vi "Send SDO.vi"() -> ()   [LabVIEW 2016]
uses:
  <vilib>/CANopenLib/CANOPEN.llb/CANopen SDO Create.vi
  <vilib>/CANopenLib/CANOPEN.llb/CANopen SDO Write [I32].vi
  <vilib>/CANopenLib/CANOPEN.llb/CANopen SDO Read [I32].vi
  <vilib>/CANopenLib/CANOPEN.llb/CANopen SDO Write [I16].vi
  <vilib>/CANopenLib/CANOPEN.llb/CANopen SDO Read [I16].vi
  <vilib>/CANopenLib/CANOPEN.llb/CANopen SDO Write [I8].vi
  <vilib>/CANopenLib/CANOPEN.llb/CANopen SDO Read [I8].vi
  <vilib>/CANopenLib/CANOPEN.llb/CANopen SDO Write [U32].vi
  <vilib>/CANopenLib/CANOPEN.llb/CANopen SDO Read [U32].vi
  <vilib>/CANopenLib/CANOPEN.llb/CANopen SDO Write [U16].vi
  <vilib>/CANopenLib/CANOPEN.llb/CANopen SDO Read [U16].vi
  <vilib>/CANopenLib/CANOPEN.llb/CANopen SDO Write [U8].vi
  <vilib>/CANopenLib/CANOPEN.llb/CANopen SDO Read [U8].vi
  <vilib>/CANopenLib/CANOPEN.llb/CANopen SDO Write [SGL].vi
  <vilib>/CANopenLib/CANOPEN.llb/CANopen SDO Read [SGL].vi
  <vilib>/CANopenLib/CANOPEN.llb/CANopen SDO Write [DBL].vi
  <vilib>/CANopenLib/CANOPEN.llb/CANopen SDO Read [DBL].vi
  <vilib>/CANopenLib/CANOPEN.llb/CANopen SDO Close.vi
  <vilib>/CANopenLib/CANOPEN.llb/CANopen Interface Close.vi
panel:
  out "error online":errorcluster
  in  "client COB-ID (0)":u32
  in  "server COB-ID (0)":u32
  in  "node-ID":u8
  out "error out":errorcluster
  in  "Blank Button 2":bool
  in  "Blank Button":bool
  in  "data":i32
  out "completion code":u32=84148224 format="%.0x"
  out "String":string
  in  "Write?":bool
  in  "object sub-index (0)":u8
  in  "object index":u16 format="%x"
  in  "Menu Ring":u16(ring) items=["u32"=3, "u8"=5]
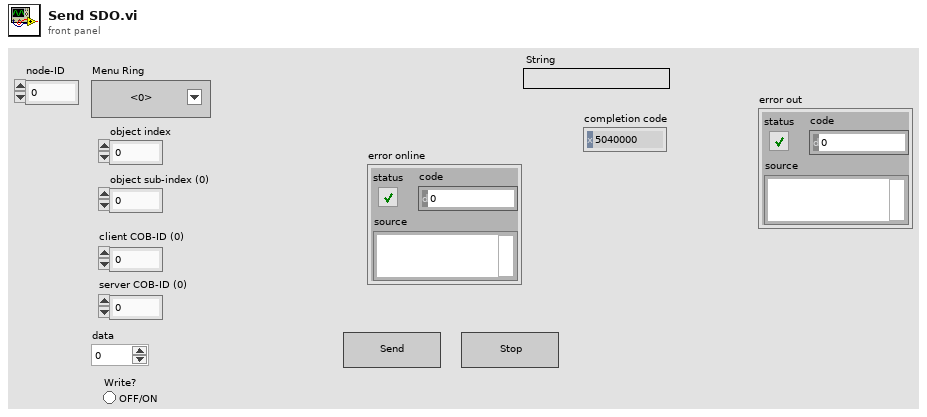
[diagram p1: front panel]
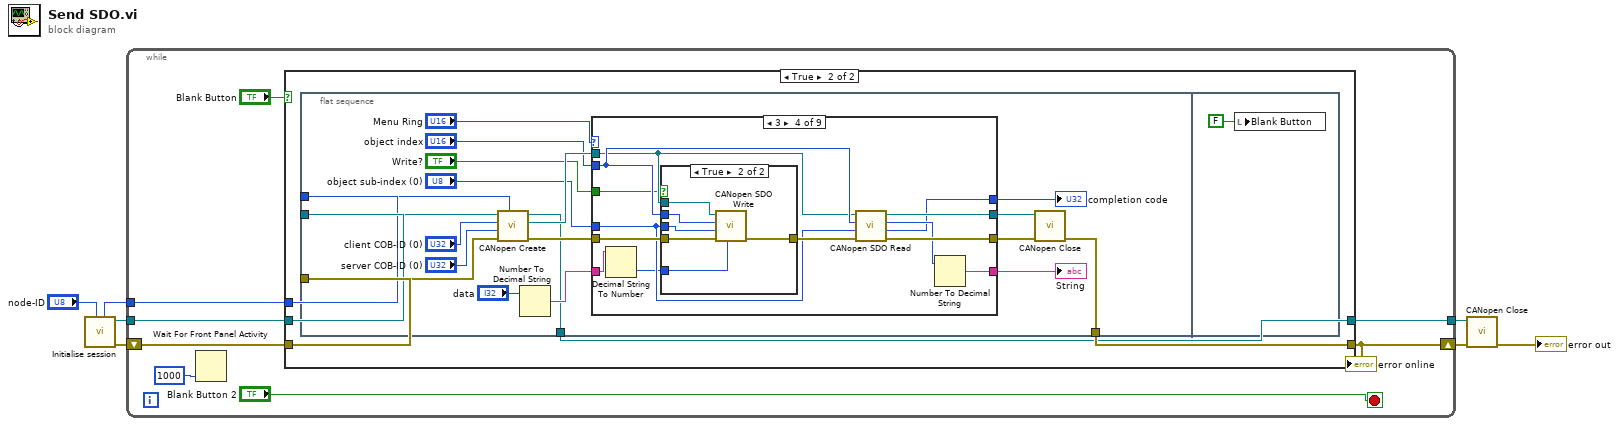
[diagram p0: block diagram]
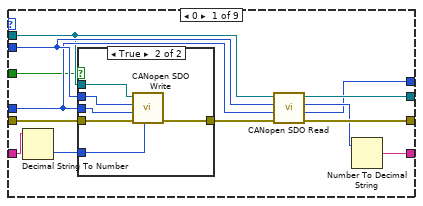
[diagram p3: hidden frame]
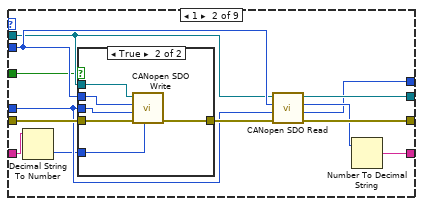
[diagram p5: hidden frame]
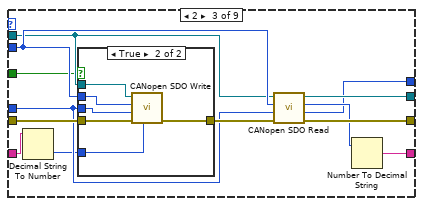
[diagram p7: hidden frame]
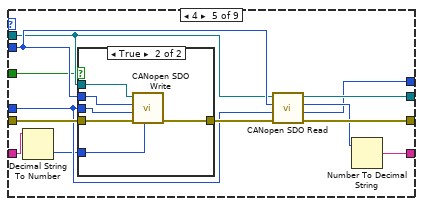
[diagram p10: hidden frame]
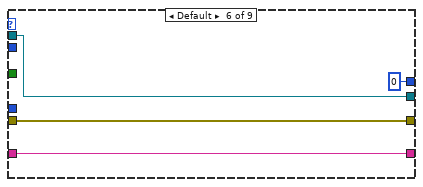
[diagram p12: hidden frame]
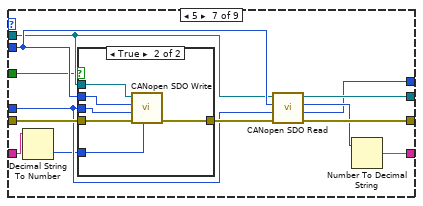
[diagram p13: hidden frame]
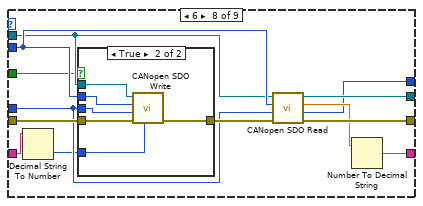
[diagram p15: hidden frame]
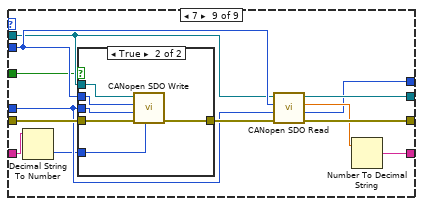
[diagram p17: hidden frame]
diagram:
  n1 = call "Initialise session.vi"("Node ID"="node-ID") -> ("error out"=w7:errorcluster, "interface object out"=w6:refnum<k20>, "Used Node ID"=w1:u8)  [unwired: 8 in]
  n2 = while {
    shift-right: [w11] -> w3
    shift-left: w7 -> [w13]
    tunnel: w6 -> [w10]
    tunnel: [w9] -> w5
    tunnel: w1 -> [w8]
    stop <- "Blank Button 2" stop-if-true
    n3 = Wait For Front Panel Activity(1:1000 ("timeout ms (-1 never timeout)")) -> ()  [unwired: 2 in, 1 out]
    n4 = case shown="True" "Blank Button" {
      tunnel: w13 -> [w16 w22]
      tunnel: [w16 w21] -> w11
      tunnel: w10 -> [w17 w20]
      tunnel: [w17 w19] -> w9
      tunnel: w8 -> [_ w18]
      frame False {
      }
      frame True {
        n5 = flat-sequence {
          tunnel: w22 -> [w29]
          tunnel: [w28] -> w21
          tunnel: w20 -> [w27]
          tunnel: [w24] -> w19
          tunnel: w18 -> [w23]
          frame #0 {
            n6 = call-poly <vilib>:"CANopen Create.vi"("node-ID"=w23, "error in (no error)"=w29, "server COB-ID (0)"="server COB-ID (0)", "client COB-ID (0)"="client COB-ID (0)", "interface object in"=w27) -> ("error out"=w41:errorcluster, "SDO object out"=w40:refnum<k20>, "interface object out"=w24:refnum<k20>)  [unwired: 4 in]
            n7 = Number To Decimal String(number="data") -> (decimal integer string=w31:string)  [unwired: 1 in]
            n8 = case shown="3" "Menu Ring" {
              tunnel: w41 -> [w54 w74 w94 w114 w134 w143 w158 w178 w198]
              tunnel: w40 -> [w48 w68 w88 w108 w128 w144 w152 w172 w192]
              tunnel: [w52 w72 w92 w112 w132 w143 w156 w176 w196] -> w39
              tunnel: [w51 w71 w91 w111 w131 w144 w155 w175 w195] -> w38
              tunnel: "object index" -> [w50 w70 w90 w110 w130 _ w154 w174 w194]
              tunnel: "object sub-index (0)" -> [w49 w69 w89 w109 w129 _ w153 w173 w193]
              tunnel: "Write?" -> [w47 w67 w87 w107 w127 _ w151 w171 w191]
              tunnel: [w46 w66 w86 w106 w126 w145 w150 w170 w190] -> w33
              tunnel: [w44 w64 w84 w104 w124 u32 0 ("completion code") w148 w168 w188] -> w32
              tunnel: w31 -> [w42 w62 w82 w102 w122 w145 w146 w166 w186]
              frame 0 {
                n9 = Decimal String To Number(string=w42) -> (number=w43:i32)  [unwired: 2 in, 1 out]
                n10 = case shown="True" w47 {
                  tunnel: w54 -> [w55 w61]
                  tunnel: w48 -> [_ w60]
                  tunnel: [w55 w59] -> w53
                  tunnel: w49 -> [_ w57]
                  tunnel: w50 -> [_ w58]
                  tunnel: w43 -> [_ w56]
                  frame False {
                  }
                  frame True {
                    n11 = call-poly <vilib>:"CANopen SDO Write.vi"("I32 data"=w56, "error in (no error)"=w61, "object sub-index (0)"=w57, "object index"=w58, "SDO object in"=w60) -> ("error out"=w59:errorcluster)  [unwired: 4 in, 2 out]
                  }
                }
                n12 = call-poly <vilib>:"CANopen SDO Read.vi"("error in (no error)"=w53, "object sub-index (0)"=w49, "object index"=w50, "SDO object in"=w48) -> ("error out"=w52:errorcluster, "completion code"=w44:u32, "I32 data"=w45:i32, "SDO object out"=w51:refnum<k20>)  [unwired: 4 in]
                n13 = Number To Decimal String(number=w45) -> (decimal integer string=w46:string)  [unwired: 1 in]
              }
              frame 1 {
                n14 = Decimal String To Number(string=w62) -> (number=w63:i32)  [unwired: 2 in, 1 out]
                n15 = case shown="True" w67 {
                  tunnel: w74 -> [w75 w81]
                  tunnel: w68 -> [_ w80]
                  tunnel: [w75 w79] -> w73
                  tunnel: w69 -> [_ w77]
                  tunnel: w70 -> [_ w78]
                  tunnel: w63 -> [_ w76]
                  frame False {
                  }
                  frame True {
                    n16 = call-poly <vilib>:"CANopen SDO Write.vi"("I16 data"=w76, "error in (no error)"=w81, "object sub-index (0)"=w77, "object index"=w78, "SDO object in"=w80) -> ("error out"=w79:errorcluster)  [unwired: 4 in, 2 out]
                  }
                }
                n17 = call-poly <vilib>:"CANopen SDO Read.vi"("error in (no error)"=w73, "object sub-index (0)"=w69, "object index"=w70, "SDO object in"=w68) -> ("error out"=w72:errorcluster, "completion code"=w64:u32, "I16 data"=w65:i16, "SDO object out"=w71:refnum<k20>)  [unwired: 4 in]
                n18 = Number To Decimal String(number=w65) -> (decimal integer string=w66:string)  [unwired: 1 in]
              }
              frame 2 {
                n19 = Decimal String To Number(string=w82) -> (number=w83:i32)  [unwired: 2 in, 1 out]
                n20 = case shown="True" w87 {
                  tunnel: w94 -> [w95 w101]
                  tunnel: w88 -> [_ w100]
                  tunnel: [w95 w99] -> w93
                  tunnel: w89 -> [_ w97]
                  tunnel: w90 -> [_ w98]
                  tunnel: w83 -> [_ w96]
                  frame False {
                  }
                  frame True {
                    n21 = call-poly <vilib>:"CANopen SDO Write.vi"("I8 data"=w96, "error in (no error)"=w101, "object sub-index (0)"=w97, "object index"=w98, "SDO object in"=w100) -> ("error out"=w99:errorcluster)  [unwired: 4 in, 2 out]
                  }
                }
                n22 = call-poly <vilib>:"CANopen SDO Read.vi"("error in (no error)"=w93, "object sub-index (0)"=w89, "object index"=w90, "SDO object in"=w88) -> ("error out"=w92:errorcluster, "completion code"=w84:u32, "I8 data"=w85:i8, "SDO object out"=w91:refnum<k20>)  [unwired: 4 in]
                n23 = Number To Decimal String(number=w85) -> (decimal integer string=w86:string)  [unwired: 1 in]
              }
              frame 3 {
                n24 = Decimal String To Number(string=w102) -> (number=w103:i32)  [unwired: 2 in, 1 out]
                n25 = case shown="True" w107 {
                  tunnel: w114 -> [w115 w121]
                  tunnel: w108 -> [_ w120]
                  tunnel: [w115 w119] -> w113
                  tunnel: w109 -> [_ w117]
                  tunnel: w110 -> [_ w118]
                  tunnel: w103 -> [_ w116]
                  frame False {
                  }
                  frame True {
                    n26 = call-poly <vilib>:"CANopen SDO Write.vi"("U32 data"=w116, "error in (no error)"=w121, "object sub-index (0)"=w117, "object index"=w118, "SDO object in"=w120) -> ("error out"=w119:errorcluster)  [unwired: 4 in, 2 out]
                  }
                }
                n27 = call-poly <vilib>:"CANopen SDO Read.vi"("error in (no error)"=w113, "object sub-index (0)"=w109, "object index"=w110, "SDO object in"=w108) -> ("error out"=w112:errorcluster, "completion code"=w104:u32, "U32 data"=w105:u32, "SDO object out"=w111:refnum<k20>)  [unwired: 4 in]
                n28 = Number To Decimal String(number=w105) -> (decimal integer string=w106:string)  [unwired: 1 in]
              }
              frame 4 {
                n29 = Decimal String To Number(string=w122) -> (number=w123:i32)  [unwired: 2 in, 1 out]
                n30 = case shown="True" w127 {
                  tunnel: w134 -> [w135 w141]
                  tunnel: w128 -> [_ w140]
                  tunnel: [w135 w139] -> w133
                  tunnel: w129 -> [_ w137]
                  tunnel: w130 -> [_ w138]
                  tunnel: w123 -> [_ w136]
                  frame False {
                  }
                  frame True {
                    n31 = call-poly <vilib>:"CANopen SDO Write.vi"("U16 data"=w136, "error in (no error)"=w141, "object sub-index (0)"=w137, "object index"=w138, "SDO object in"=w140) -> ("error out"=w139:errorcluster)  [unwired: 4 in, 2 out]
                  }
                }
                n32 = call-poly <vilib>:"CANopen SDO Read.vi"("error in (no error)"=w133, "object sub-index (0)"=w129, "object index"=w130, "SDO object in"=w128) -> ("error out"=w132:errorcluster, "completion code"=w124:u32, "U16 data"=w125:u16, "SDO object out"=w131:refnum<k20>)  [unwired: 4 in]
                n33 = Number To Decimal String(number=w125) -> (decimal integer string=w126:string)  [unwired: 1 in]
              }
              frame Default {
              }
              frame 5 {
                n34 = Decimal String To Number(string=w146) -> (number=w147:i32)  [unwired: 2 in, 1 out]
                n35 = case shown="True" w151 {
                  tunnel: w158 -> [w159 w165]
                  tunnel: w152 -> [_ w164]
                  tunnel: [w159 w163] -> w157
                  tunnel: w153 -> [_ w161]
                  tunnel: w154 -> [_ w162]
                  tunnel: w147 -> [_ w160]
                  frame False {
                  }
                  frame True {
                    n36 = call-poly <vilib>:"CANopen SDO Write.vi"("U8 data"=w160, "error in (no error)"=w165, "object sub-index (0)"=w161, "object index"=w162, "SDO object in"=w164) -> ("error out"=w163:errorcluster)  [unwired: 4 in, 2 out]
                  }
                }
                n37 = call-poly <vilib>:"CANopen SDO Read.vi"("error in (no error)"=w157, "object sub-index (0)"=w153, "object index"=w154, "SDO object in"=w152) -> ("error out"=w156:errorcluster, "completion code"=w148:u32, "U8 data"=w149:u8, "SDO object out"=w155:refnum<k20>)  [unwired: 4 in]
                n38 = Number To Decimal String(number=w149) -> (decimal integer string=w150:string)  [unwired: 1 in]
              }
              frame 6 {
                n39 = Decimal String To Number(string=w166) -> (number=w167:i32)  [unwired: 2 in, 1 out]
                n40 = case shown="True" w171 {
                  tunnel: w178 -> [w179 w185]
                  tunnel: w172 -> [_ w184]
                  tunnel: [w179 w183] -> w177
                  tunnel: w173 -> [_ w181]
                  tunnel: w174 -> [_ w182]
                  tunnel: w167 -> [_ w180]
                  frame False {
                  }
                  frame True {
                    n41 = call-poly <vilib>:"CANopen SDO Write.vi"("SGL data"=w180, "error in (no error)"=w185, "object sub-index (0)"=w181, "object index"=w182, "SDO object in"=w184) -> ("error out"=w183:errorcluster)  [unwired: 4 in, 2 out]
                  }
                }
                n42 = call-poly <vilib>:"CANopen SDO Read.vi"("error in (no error)"=w177, "object sub-index (0)"=w173, "object index"=w174, "SDO object in"=w172) -> ("error out"=w176:errorcluster, "completion code"=w168:u32, "SGL data"=w169:sgl, "SDO object out"=w175:refnum<k20>)  [unwired: 4 in]
                n43 = Number To Decimal String(number=w169) -> (decimal integer string=w170:string)  [unwired: 1 in]
              }
              frame 7 {
                n44 = Decimal String To Number(string=w186) -> (number=w187:i32)  [unwired: 2 in, 1 out]
                n45 = case shown="True" w191 {
                  tunnel: w198 -> [w199 w205]
                  tunnel: w192 -> [_ w204]
                  tunnel: [w199 w203] -> w197
                  tunnel: w193 -> [_ w201]
                  tunnel: w194 -> [_ w202]
                  tunnel: w187 -> [_ w200]
                  frame False {
                  }
                  frame True {
                    n46 = call-poly <vilib>:"CANopen SDO Write.vi"("DBL data"=w200, "error in (no error)"=w205, "object sub-index (0)"=w201, "object index"=w202, "SDO object in"=w204) -> ("error out"=w203:errorcluster)  [unwired: 4 in, 2 out]
                  }
                }
                n47 = call-poly <vilib>:"CANopen SDO Read.vi"("error in (no error)"=w197, "object sub-index (0)"=w193, "object index"=w194, "SDO object in"=w192) -> ("error out"=w196:errorcluster, "completion code"=w188:u32, "DBL data"=w189:dbl, "SDO object out"=w195:refnum<k20>)  [unwired: 4 in]
                n48 = Number To Decimal String(number=w189) -> (decimal integer string=w190:string)  [unwired: 1 in]
              }
            }
            "String" <- w33
            "completion code" <- w32
            n49 = call-poly <vilib>:"CANopen Close.vi"("error in (no error)"=w39, "SDO object in"=w38) -> ("error out"=w28:errorcluster)  [unwired: 9 in]
          }
          frame #1 {
            n50 = local write "Blank Button"(FALSE) -> ()
          }
        }
      }
    }
    "error online" <- w11
  }
  n51 = call-poly <vilib>:"CANopen Close.vi"("error in (no error)"=w3, "interface object in"=w5) -> ("error out"=→"error out":errorcluster)  [unwired: 9 in]
